vi "Test cells.vi"(11 "Test Case In":refnum<class "Test Cases.lvclass">) -> (0 "error out":errorcluster, 3 "Test Case Out":refnum<class "Test Cases.lvclass">)   [LabVIEW 2024, in "Test Cases.lvclass"]
uses:
  Test Cases.lvclass
  C:/Program Files/National Instruments/LabVIEW 2025/vi.lib/Astemes/LUnit/Test Case.lvclass
  D:/git/Sourcegrid-LabVIEW/dll/SourceGrid.dll
  dll/SourceGrid.dll
  source/Grid/SourceGrid.lvclass
  source/Cells/Image/Image.lvclass
  D:/git/Sourcegrid-LabVIEW/source/Cells/Cell/Cell.lvclass
  <vilib>/Astemes/LUnit/Test Case.lvclass/Test Case.ctl
  <vilib>/Astemes/LUnit/Append Pass Result.vi
  <vilib>/Astemes/LUnit/Append Fail Result.vi
  <vilib>/Astemes/LUnit/Run In UI.vi
  <vilib>/Utility/error.llb/Clear Errors.vi
  source/Grid/Set Column Default Width.vi
  <vilib>/Astemes/LUnit/Test Case.lvclass
  source/Cells/Cell/Cell.lvclass
panel:
  in  "stop":bool
  in  "Grid Container":refnum<k24>(container)
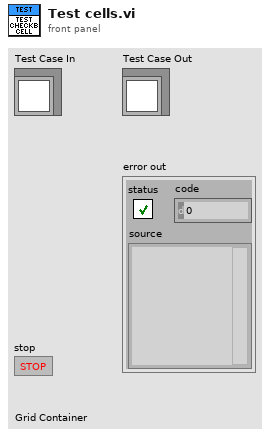
[diagram p1: front panel]
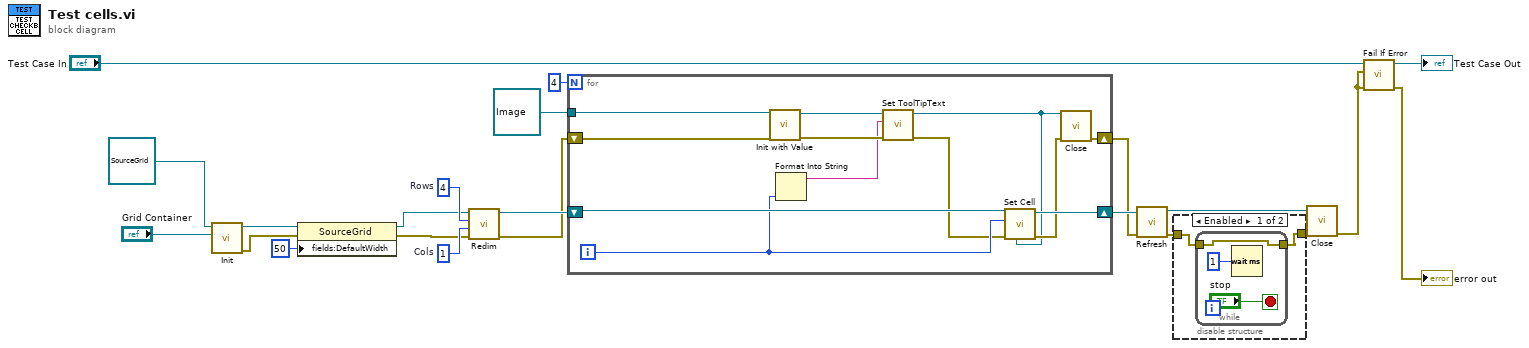
[diagram p0: block diagram]
diagram:
  w18 = 1  # Cols
  w19 = 4  # Rows
  n1 = call-dynamic "Init.vi"("Sourcegrid Container"="Grid Container", "Grid in"=refnum<class "SourceGrid.lvclass"> refnum) -> ("error out"=w6:errorcluster, "Grid out"=w15:refnum<class "SourceGrid.lvclass">)  [unwired: 8 in]
  n2 = property class="SourceGrid"(reference=w15, error in=w6, "fields:DefaultWidth"=50 ("DefaultWidth")) -> (reference out=w14:refnum<class "SourceGrid.lvclass">, error out=w13:errorcluster)
  n3 = call "Redim.vi"("error in"=w13, "Columns"=w18, "Rows"=w19, "Sourcegrid in"=w14) -> ("error out"=w1:errorcluster, "Sourcegrid out"=w10:refnum<class "SourceGrid.lvclass">)  [unwired: 6 in]
  n4 = for {
    N: 4 -> [_]
    shift-right: [w32] -> w2
    shift-left: w1 -> [w29]
    shift-right: [w34] -> w11
    shift-left: w10 -> [w33]
    tunnel: refnum<class "Image.lvclass"> refnum ("Cell in") -> [w30]
    i -> [w26]
    n5 = call-dynamic "Init with Value.vi"("error in"=w29, "Image in"=w30) -> ("error out"=w28:errorcluster, "Image out"=w27:refnum<class "Image.lvclass">)  [unwired: 8 in]
    n6 = Format Into String(w26) -> (resulting string=w25:string)  [unwired: 3 in, 1 out]
    n7 = call "Set ToolTipText.vi"("error in"=w28, "ToolTipText"=w25, "Cell in"=w27) -> ("error out"=w24:errorcluster, "Cell out"=w23:refnum<class "Image.lvclass">)  [unwired: 7 in]
    n8 = call "Set Cell.vi"("Cell"=w23, "error in"=w24, "Row"=w26, "Sourcegrid in"=w33) -> ("error out"=w31:errorcluster, "Sourcegrid out"=w34:refnum<class "SourceGrid.lvclass">)  [unwired: 6 in]
    n9 = call-dynamic "Close.vi"("error in"=w31, "Cell in"=w23) -> ("error out"=w32:errorcluster)  [unwired: 8 in, 1 out]
  }
  n10 = call "Refresh.vi"("error in"=w2, "SourceGrid in"=w11) -> ("error out"=w4:errorcluster, "SourceGrid out"=w8:refnum<class "SourceGrid.lvclass">)  [unwired: 8 in]
  n11 = disable-structure shown="Enabled" {
    disable-tunnel: w4 -> [w36 w40]
    disable-tunnel: [w35 w40] -> w3
    frame Enabled {
      n12 = while {
        tunnel: w36 -> [w37]
        tunnel: [w37] -> w35
        stop <- "stop" stop-if-true
        n13 = Wait (ms)(milliseconds to wait=u32 1) -> ()  [unwired: 1 out]
      }
    }
    frame Disabled {
    }
  }
  n14 = call-dynamic "Close.vi"("error in"=w3, "Sourcegrid in"=w8) -> ("error out"=w17:errorcluster)  [unwired: 8 in, 1 out]
  n15 = call <vilib>:"Fail If Error.vi"("error in (no error)"=w17, "Assert error"=w17, "LUnit Test Case In"="Test Case In") -> ("error out"=→"error out":errorcluster, "LUnit Test Case Out"=→"Test Case Out":refnum<class "Test Cases.lvclass">)  [unwired: 7 in]
